vi "inverse tan 0to359.vi"(10 "y coil":dbl=1e-05 format="%#_13g", 11 "z coil":dbl format="%#_13g") -> (3 "phi (deg)":dbl format="%#_5f")   [LabVIEW 2013]
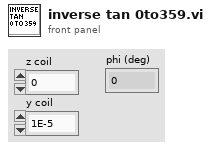
[diagram p1: front panel]
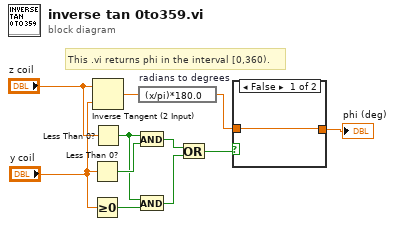
[diagram p0: block diagram]
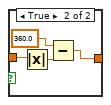
[diagram p2: hidden frame]
diagram:
  # "This .vi returns phi in the interval [0,360)."
  n1 = Less Than 0?(x="y coil") -> (x < 0?=w9:bool)
  n2 = Greater Or Equal To 0?(x="y coil") -> (x >= 0?=w2:bool)
  n3 = Inverse Tangent (2 Input)(1:"y coil", 2:"z coil") -> (0:w11:dbl)
  n4 = Less Than 0?(x="z coil") -> (x < 0?=w3:bool)
  n5 = And(x=w3, y=w9) -> (x .and. y?=w6:bool)
  n6 = And(x=w3, y=w2) -> (x .and. y?=w5:bool)
  n7 = expression code="(x/pi)*180.0" "radians to degrees"(w11) -> (w8:dbl)
  n8 = Or(x=w6, y=w5) -> (x .or. y?=w4:bool)
  n9 = case shown="False" w4 {
    tunnel: w8 -> [w12 w16]
    tunnel: [w12 w13] -> w7
    frame False {
    }
    frame True {
      n10 = Absolute Value(x=w16) -> (abs(x)=w15:dbl)
      n11 = Subtract(x=360.0, y=w15) -> (x-y=w13:dbl)
    }
  }
  "phi (deg)" <- w7
